vi "WaitTillStop.vi"() -> (0 "Error Status":bool, 1 "Stopped":bool)   [LabVIEW 2022 SP3]
uses:
  Power ON_OFF.vi
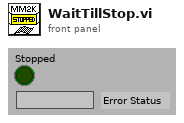
[diagram p1: front panel]
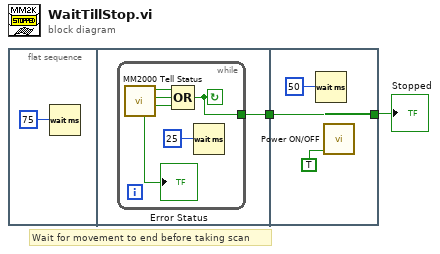
[diagram p0: block diagram]
diagram:
  # "Wait for movement to end before taking scan"
  n1 = flat-sequence {
    tunnel: [w4] -> w1
    tunnel: [w13] -> w2
    tunnel: w1 -> [w13]
    frame #0 {
      n2 = Wait (ms)(milliseconds to wait=75) -> ()  [unwired: 1 out]
    }
    frame #1 {
      n3 = while {
        tunnel: [w6] -> w4
        stop <- w6 continue-if-true
        n4 = call "MM2000 Tell Status.vi"() -> ("Error Status"=→"Error Status":bool, "Axis1 Status"=w10:bool, "Axis2 Status"=w9:bool, "Axis3 Status"=w8:bool)  [unwired: 1 in, 3 out]
        n5 = Compound Arithmetic op=OR(w10, w9, w8) -> (w6:bool)
        n6 = Wait (ms)(milliseconds to wait=25) -> ()  [unwired: 1 out]
      }
    }
    frame #2 {
      n7 = Wait (ms)(milliseconds to wait=50) -> ()  [unwired: 1 out]
      n8 = call "Power ON/OFF.vi"("OFF (T)/ON (F)"=TRUE) -> ()  [unwired: 4 in, 1 out]
    }
  }
  "Stopped" <- w2
